vi "CanSatDashboard.vi"() -> ()   [LabVIEW 2018]
uses:
  <vilib>/Instr/_visa.llb/VISA Configure Serial Port (Instr).vi
panel:
  in  "stop":bool
  out "Giroscopio Z":dbl format="%#_6f"
  out "Giroscopio Y":dbl format="%#_6f"
  out "Acelerómetro Z":dbl
  out "Acelerómetro Y":dbl
  out "Magnetometro Z":dbl
  out "Magnetometro Y":dbl
  out "Humedad":dbl(slide) scale=0.0..1023.0
  out "Longitud":dbl
  out "Nivel de Batería":dbl(slide) scale=0.0..100.0
  out "Giroscopio X":dbl format="%#_6f"
  out "C4H10":dbl(slide) scale=0.0..1023.0
  out "NO2":dbl(slide) scale=0.0..1023.0
  out "NH3":dbl(slide) scale=0.0..1023.0
  out "Temperatura Ext.":dbl(slide) scale=0.0..60.0
  out "H2":dbl(slide) scale=0.0..1023.0
  out "UV":dbl(slide) scale=0.0..1023.0
  out "Latitud":dbl
  out "Acelerómetro X":dbl
  out "Magnetometro X":dbl
  out "Barómetro":dbl(knob) scale=0.0..1000000.0
  out "PM":dbl
  out "C2H5OH":dbl(slide) scale=0.0..1023.0
  out "Metano":dbl(slide) scale=0.0..1023.0
  out "C3H8":dbl(slide) scale=0.0..1023.0
  out "CO":dbl(slide) scale=0.0..1023.0
  out "Temeperatura Int.":dbl(slide) scale=0.0..100.0
  out "Valor":string
  in  "VISA":refnum<visa-resource-name>
  # "CanSat Dashboard"
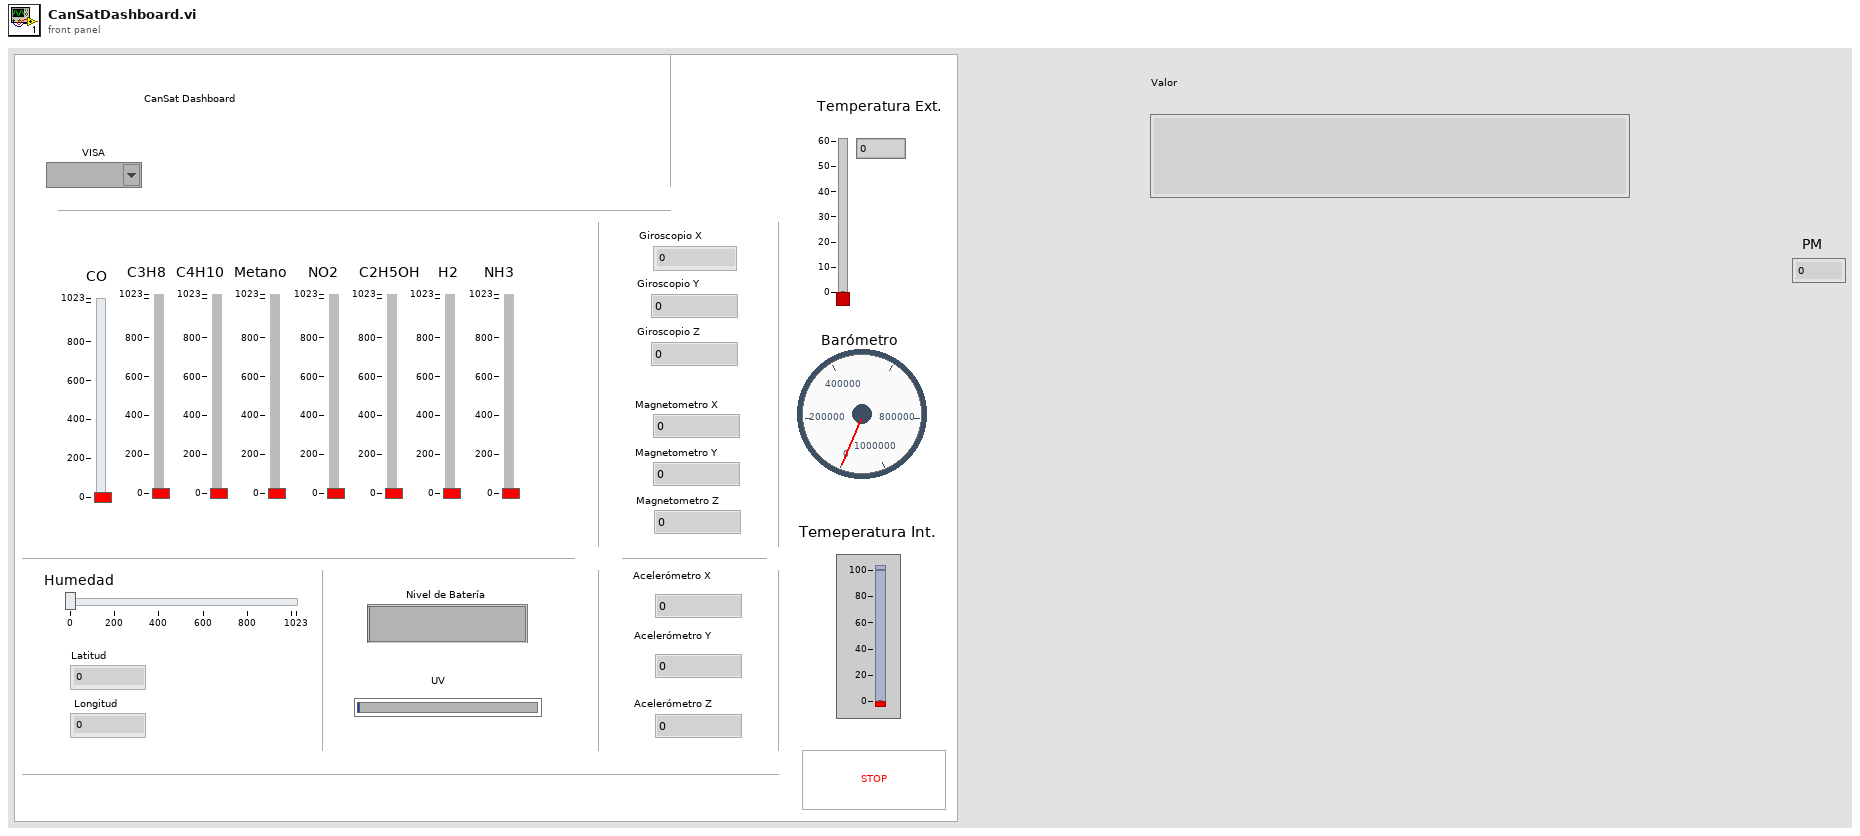
[diagram p1: front panel]
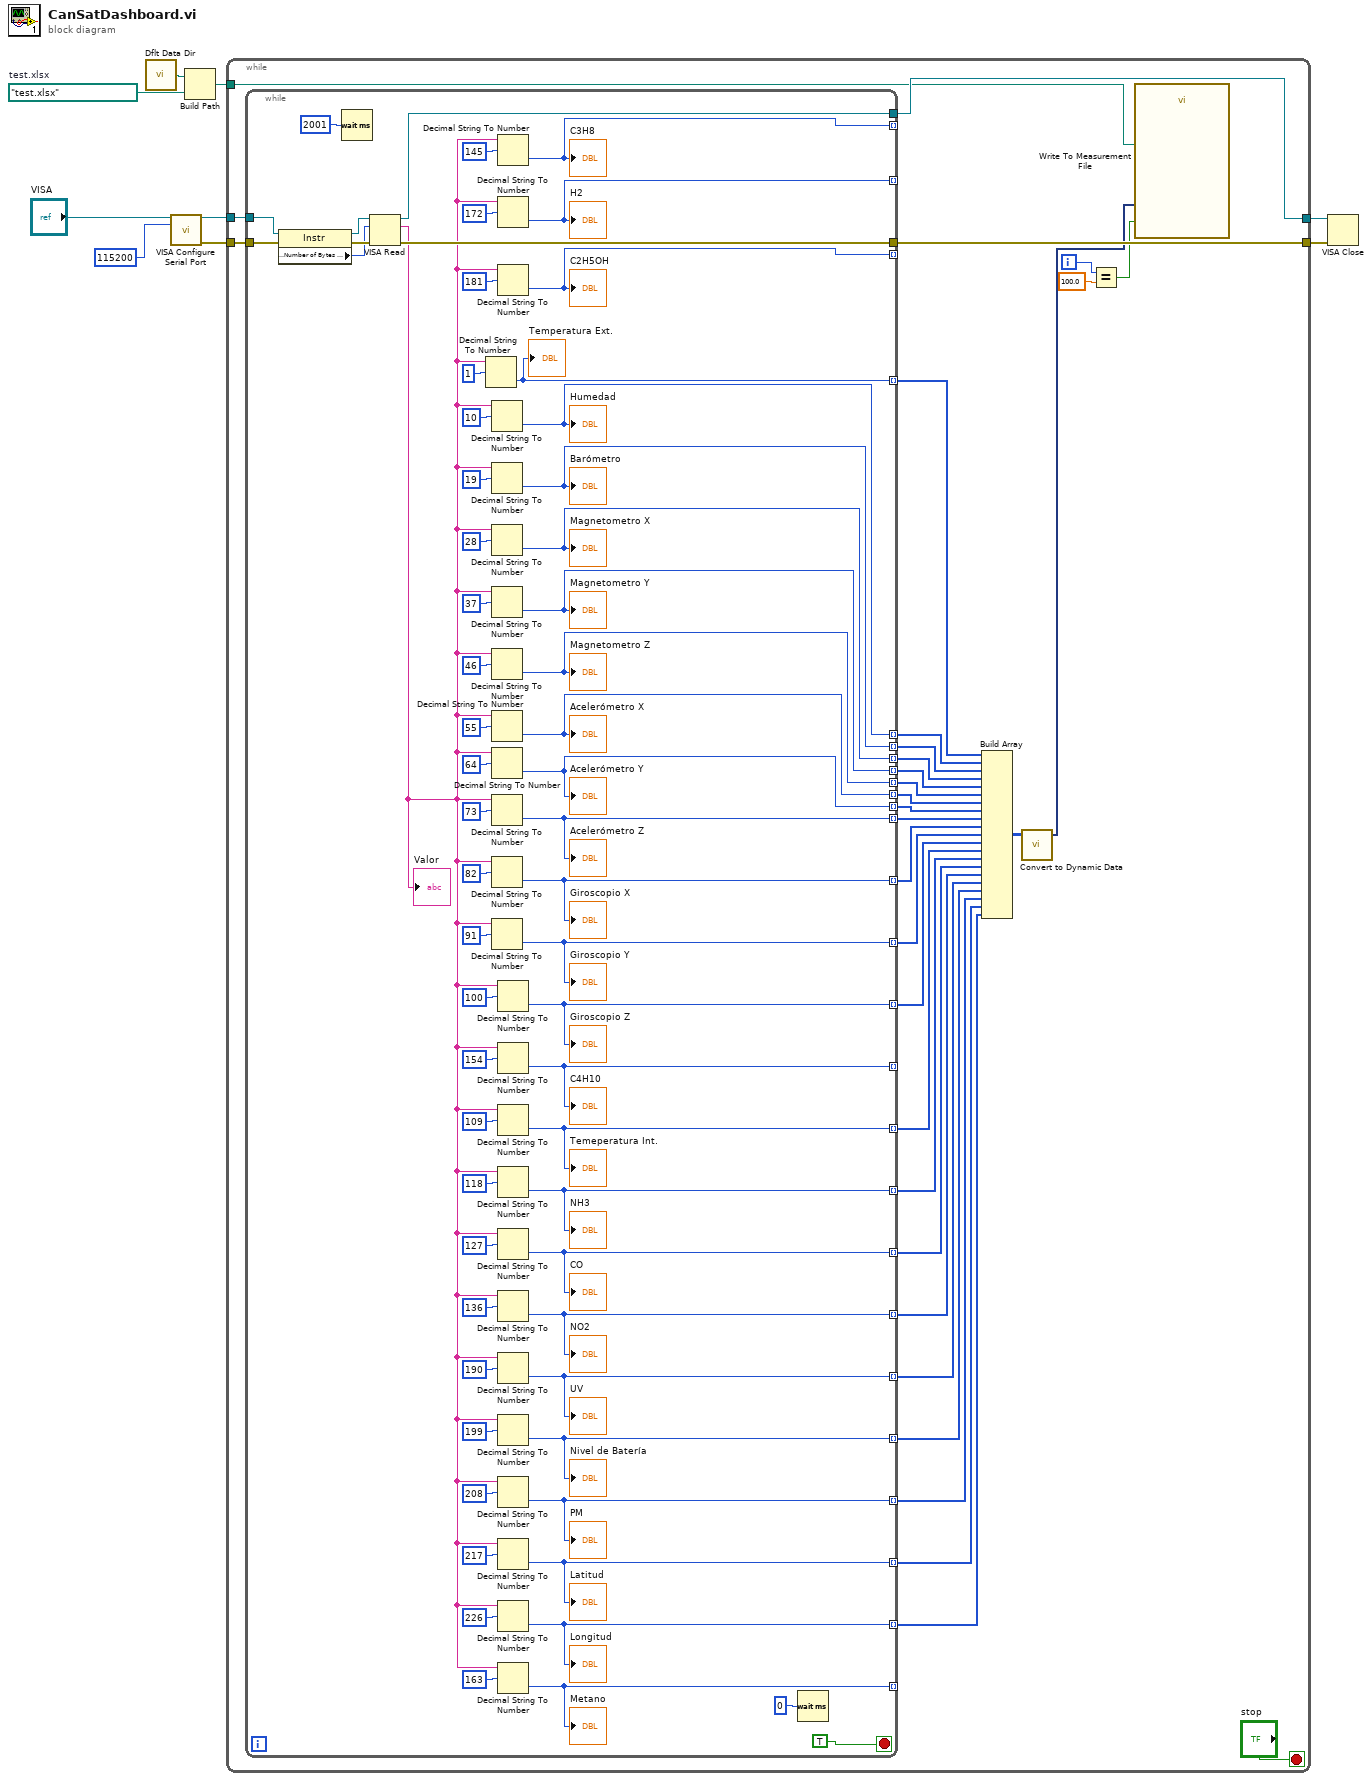
[diagram p0: block diagram]
diagram:
  w2 = path "test.xlsx"  # test.xlsx
  n1 = call <vilib>:"Dflt Data Dir.vi"() -> ("App:Default Data Directory"=w3:path)
  n2 = call-poly "VISA Configure Serial Port"("VISA resource name"="VISA", "baud rate (9600)"=u32 115200) -> ("VISA resource name out"=w9:refnum<visa-resource-name>, "error out"=w8:errorcluster)  [unwired: 12 in]
  n3 = Build Path(base path=w3, name or relative path=w2) -> (appended path=w1:path)
  n4 = while {
    tunnel: w9 -> [w41]
    tunnel: w8 -> [w40]
    tunnel: [w39] -> w5
    tunnel: [w38] -> w4
    tunnel: w1 -> [w12]
    i -> [w11]
    stop <- "stop" stop-if-true
    n5 = while {
      tunnel: w41 -> [w104]
      tunnel: [w102] -> w38
      tunnel: w40 -> [w101]
      tunnel: [w99] -> w39
      tunnel: [w68] -> w36 mode=indexing
      tunnel: [w67] -> w37 mode=indexing
      tunnel: [w66] -> w35 mode=indexing
      tunnel: [w65] -> w34 mode=indexing
      tunnel: [w64] -> w33 mode=indexing
      tunnel: [w63] -> w32 mode=indexing
      tunnel: [w62] -> w31 mode=indexing
      tunnel: [w61] -> w30 mode=indexing
      tunnel: [w60] -> w29 mode=indexing
      tunnel: [w59] -> w28 mode=indexing
      tunnel: [w58] -> w27 mode=indexing
      tunnel: [w57] -> w26 mode=indexing
      tunnel: [w56] -> w25 mode=indexing
      tunnel: [w55] -> w24 mode=indexing
      tunnel: [w54] -> w23 mode=indexing
      tunnel: [w53] -> w22 mode=indexing
      tunnel: [w52] -> _ mode=indexing
      tunnel: [w51] -> _ mode=indexing
      tunnel: [w50] -> _ mode=indexing
      tunnel: [w49] -> _ mode=indexing
      tunnel: [w48] -> _ mode=indexing
      tunnel: [w47] -> w21 mode=indexing
      tunnel: [w46] -> w20 mode=indexing
      tunnel: [w45] -> w19 mode=indexing
      tunnel: [w44] -> w18 mode=indexing
      tunnel: [w43] -> w17 mode=indexing
      stop <- TRUE stop-if-true
      n6 = property class="Instr"(reference=w104, error in=w101) -> (reference out=w103:refnum<visa-resource-name>, error out=w100:errorcluster, "Serial Settings:Number of Bytes at Serial Port"=w87:u32)
      n7 = Wait (ms)(milliseconds to wait=u32 2001) -> ()  [unwired: 1 out]
      n8 = VISA Read(VISA resource name=w103, byte count=w87, error in (no error)=w100) -> (VISA resource name out=w102:refnum<visa-resource-name>, read buffer=w69:string, error out=w99:errorcluster)  [unwired: 1 out]
      "Valor" <- w69
      n9 = Decimal String To Number(string=w69, offset=1) -> (number=w68:i32)  [unwired: 1 in, 1 out]
      "Temperatura Ext." <- w68
      n10 = Decimal String To Number(string=w69, offset=10) -> (number=w67:i32)  [unwired: 1 in, 1 out]
      "Humedad" <- w67
      n11 = Decimal String To Number(string=w69, offset=19) -> (number=w66:i32)  [unwired: 1 in, 1 out]
      "Barómetro" <- w66
      n12 = Decimal String To Number(string=w69, offset=28) -> (number=w65:i32)  [unwired: 1 in, 1 out]
      "Magnetometro X" <- w65
      n13 = Decimal String To Number(string=w69, offset=37) -> (number=w64:i32)  [unwired: 1 in, 1 out]
      "Magnetometro Y" <- w64
      n14 = Decimal String To Number(string=w69, offset=46) -> (number=w63:i32)  [unwired: 1 in, 1 out]
      "Magnetometro Z" <- w63
      n15 = Decimal String To Number(string=w69, offset=55) -> (number=w62:i32)  [unwired: 1 in, 1 out]
      "Acelerómetro X" <- w62
      n16 = Decimal String To Number(string=w69, offset=64) -> (number=w61:i32)  [unwired: 1 in, 1 out]
      "Acelerómetro Y" <- w61
      n17 = Decimal String To Number(string=w69, offset=73) -> (number=w60:i32)  [unwired: 1 in, 1 out]
      "Acelerómetro Z" <- w60
      n18 = Decimal String To Number(string=w69, offset=82) -> (number=w59:i32)  [unwired: 1 in, 1 out]
      "Giroscopio X" <- w59
      n19 = Decimal String To Number(string=w69, offset=91) -> (number=w58:i32)  [unwired: 1 in, 1 out]
      "Giroscopio Y" <- w58
      n20 = Decimal String To Number(string=w69, offset=145) -> (number=w52:i32)  [unwired: 1 in, 1 out]
      "C3H8" <- w52
      n21 = Decimal String To Number(string=w69, offset=172) -> (number=w49:i32)  [unwired: 1 in, 1 out]
      "H2" <- w49
      n22 = Decimal String To Number(string=w69, offset=181) -> (number=w48:i32)  [unwired: 1 in, 1 out]
      "C2H5OH" <- w48
      n23 = Decimal String To Number(string=w69, offset=100) -> (number=w57:i32)  [unwired: 1 in, 1 out]
      "Giroscopio Z" <- w57
      n24 = Decimal String To Number(string=w69, offset=154) -> (number=w51:i32)  [unwired: 1 in, 1 out]
      "C4H10" <- w51
      n25 = Decimal String To Number(string=w69, offset=109) -> (number=w56:i32)  [unwired: 1 in, 1 out]
      "Temeperatura Int." <- w56
      n26 = Decimal String To Number(string=w69, offset=118) -> (number=w55:i32)  [unwired: 1 in, 1 out]
      "NH3" <- w55
      n27 = Decimal String To Number(string=w69, offset=127) -> (number=w54:i32)  [unwired: 1 in, 1 out]
      "CO" <- w54
      n28 = Decimal String To Number(string=w69, offset=136) -> (number=w53:i32)  [unwired: 1 in, 1 out]
      "NO2" <- w53
      n29 = Decimal String To Number(string=w69, offset=190) -> (number=w47:i32)  [unwired: 1 in, 1 out]
      "UV" <- w47
      n30 = Decimal String To Number(string=w69, offset=199) -> (number=w46:i32)  [unwired: 1 in, 1 out]
      "Nivel de Batería" <- w46
      n31 = Decimal String To Number(string=w69, offset=208) -> (number=w45:i32)  [unwired: 1 in, 1 out]
      "PM" <- w45
      n32 = Decimal String To Number(string=w69, offset=217) -> (number=w44:i32)  [unwired: 1 in, 1 out]
      "Latitud" <- w44
      n33 = Decimal String To Number(string=w69, offset=226) -> (number=w43:i32)  [unwired: 1 in, 1 out]
      "Longitud" <- w43
      n34 = Decimal String To Number(string=w69, offset=163) -> (number=w50:i32)  [unwired: 1 in, 1 out]
      "Metano" <- w50
      n35 = Wait (ms)(milliseconds to wait=u32 0) -> ()  [unwired: 1 out]
    }
    n36 = Build Array(w36, w37, w35, w34, w33, w32, w31, w30, w29, w28, w27, w26, w25, w24, w23, w22, w21, w20, w19, w18, w17) -> (w13:i32[][])
    n37 = call "Convert to Dynamic Data"("2D Array"=w13) -> ("Dynamic Data Type"=w16:dynamicdata)  [unwired: 3 in]
    n38 = Equal?(x=w11, y=100.0) -> (x = y?=w14:bool)
    n39 = call "Write To Measurement File"("Signals"=w16, "Flush? (T)"=w14, "Filename"=w12) -> ()  [unwired: 14 in, 3 out]
  }
  n40 = VISA Close(VISA resource name=w4, error in (no error)=w5) -> ()  [unwired: 1 out]
